vi "Flush Pretrigger Data Buffer.vi"(8 "error in (no error)":errorcluster, 11 "Triggered Log in":refnum<class "Triggered Log.lvclass">) -> (0 "error out":errorcluster, 3 "Triggered Log out":refnum<class "Triggered Log.lvclass">)   [LabVIEW 2012, in "Triggered Log.lvclass"]
doc: "Flushes any data in the pretrigger data buffer to the active log file instance. Updates the triggered log state if the underlying segmented log completes."
uses:
  Triggered Log.lvclass
  Triggered Log.lvclass/Triggered Log.ctl
  Engine/Classes/Logs/Segmented Logs/Segmented Log/Segmented Log.lvclass/Segmented Log.ctl
  Shared/Classes/Log File Specifications/Log File Specification/Log File Specification.lvclass/Log File Specification.ctl
  Triggered Log State.ctl
  Flush Buffer Data.vi
  Engine/Classes/Logs/Segmented Logs/Segmented Log/Write Data to Log File Instance (Waveform).vi
  Engine/Classes/Logs/Segmented Logs/Segmented Log/Write Data to Log File Instance.vi
  On Triggered Log State Change.vi
  Engine/Classes/Logs/Segmented Logs/Segmented Log/Check Close File.vi
  Engine/Classes/Logs/Segmented Logs/Segmented Log/Check Open File.vi
  Engine/Classes/Logs/Segmented Logs/Segmented Log/Close Log File Instance.vi
  Engine/Classes/Logs/Segmented Logs/Segmented Log/Open Log File Instance.vi
  Engine/Classes/Logs/Segmented Logs/Segmented Log/On Segmented Log Complete.vi
  Engine/Classes/Logs/Segmented Logs/Segmented Log/On File Close.vi
  Shared/Classes/Log File Specifications/Log File Specification/Open Log File.vi
  Shared/Classes/Log File Specifications/Log File Specification/Set Path Tag.vi
  Engine/Classes/Logs/Segmented Logs/Segmented Log/On File Open.vi
  Shared/Classes/Log File Specifications/Log File Specification/Set Filename Offset.vi
  Shared/Classes/Log File Specifications/Log File Specification/Build File Path.vi
  Shared/Classes/Log File Specifications/Log File Specification/Resolve File Conflicts.vi
  Shared/Classes/Log File Specifications/Log File Specification/Initialize Log File.vi
  <vilib>/Utility/libraryn.llb/Check if File or Folder Exists.vi
  <vilib>/Utility/error.llb/Error Cluster From Error Code.vi
  <vilib>/Utility/libraryn.llb/Get File Extension.vi
  <vilib>/Utility/libraryn.llb/Create Directory Recursive.vi
  Engine/Classes/Logs/Log Files/Log File/Write to Log File (Waveform).vi
  Engine/Classes/Logs/Segmented Logs/Segmented Log/Segment Log File.vi
  Engine/Classes/Logs/Log Files/Log File/Close Log File.vi
  Engine/Classes/Logs/Segmented Logs/Segmented Log/Make File Read-Only.vi
  Engine/Classes/Logs/Log Files/Log File/Write to Log File.vi
  Engine/Classes/Triggers/Trigger/Finalize.vi
  Engine/Classes/Logs/Log Files/Log File/Log File.lvclass
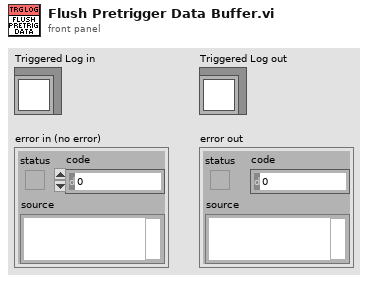
[diagram p1: front panel]
types:
  T1 = typedef "Triggered Log.lvclass/Triggered Log State.ctl" = enum16{"Waiting on Trigger", "Triggered", "Posttrigger", "Complete", "Idle", "Error"}
  T2 = typedef "Triggered Log.lvclass/Buffer Data.ctl" = cluster{"Position":i32, "Length":i32, "Max Length":i32, "Channel Count":i32, "Data":dbl[][], "t0 Array":timestamp[]}
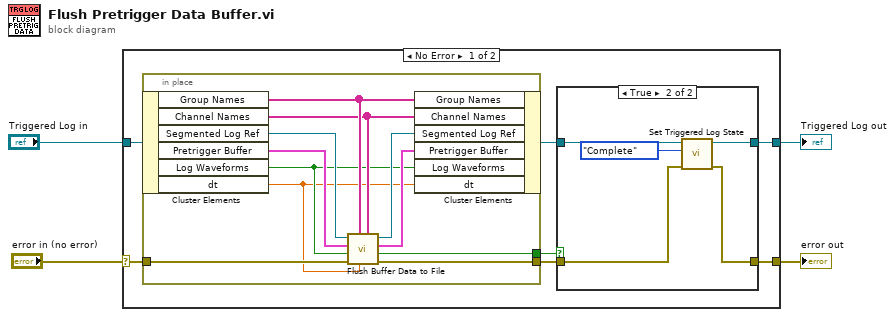
[diagram p0: block diagram]
diagram:
  n1 = case shown="No Error" "error in (no error)" {
    selector: "error in (no error)" -> [w5 w30]
    tunnel: "Triggered Log in" -> [w11 w31]
    tunnel: [w8 w31] -> w3
    tunnel: [w7 w30] -> w2
    frame No Error {
      n2 = in-place {
        in-place-border: w5 -> [w29]
        in-place-border: [w28] -> w9
        in-place-border: [w21] -> w6
        n3 = in-place-cluster #1(w11) -> ("Group Names"=w25:string[], "Channel Names"=w24:string[], "Segmented Log Ref"=w27:refnum<data-value>, "Pretrigger Buffer"=w23:T2, "Log Waveforms"=w20:bool, "dt"=w19:dbl)
        n4 = call "Flush Buffer Data to File.vi"("Channel Names"=w24, "dt"=w19, "Group Names"=w25, "error in (no error)"=w29, "Waveform"=w20, "Buffer Data in"=w23, "Segmented Log Ref in"=w27) -> ("error out"=w28:errorcluster, "Log Completed"=w21:bool, "Buffer Data out"=w22:T2, "Segmented Log Ref out"=w26:refnum<data-value>)  [unwired: 1 in]
        n5 = in-place-cluster #1("Group Names"=w25, "Channel Names"=w24, "Segmented Log Ref"=w26, "Pretrigger Buffer"=w22, "Log Waveforms"=w20, "dt"=w19) -> (w10:refnum<class "Triggered Log.lvclass">)
      }
      n6 = case shown="True" w6 {
        tunnel: w9 -> [w12 w18]
        tunnel: [w12 w17] -> w7
        tunnel: [w13 w16] -> w8
        tunnel: w10 -> [w13 w15]
        frame False {
        }
        frame True {
          n7 = call "Set Triggered Log State.vi"("error in (no error)"=w18, "Triggered Log State"=Triggered_Log_State."Complete", "Triggered Log in"=w15) -> ("error out"=w17:errorcluster, "Triggered Log out"=w16:refnum<class "Triggered Log.lvclass">)  [unwired: 7 in]
        }
      }
    }
    frame Error {
    }
  }
  "Triggered Log out" <- w3
  "error out" <- w2
